vi "Pause.vi"(8 "error in (no error)":errorcluster, 11 "VICI Settings":T1) -> (0 "error out":errorcluster, 1 "Connection Error":bool, 3 "VICI Settings":T1)   [LabVIEW 2018, in "VICI M50 Party Mode.lvlib"]
uses:
  VICI M50 Party Mode.lvlib
  Settings Cluster.ctl
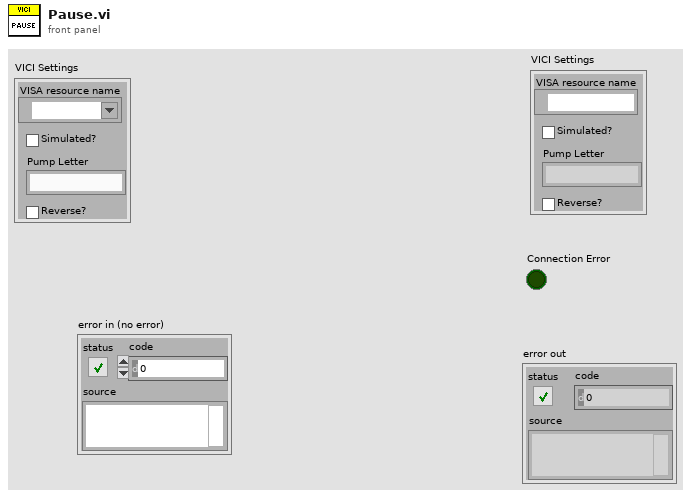
[diagram p1: front panel]
types:
  T1 = typedef "VICI M50 Party Mode.lvlib/Settings Cluster.ctl" = cluster{"VISA resource name":refnum<visa-resource-name>, "Simulated?":bool, "Pump Letter":string, "Reverse?":bool}
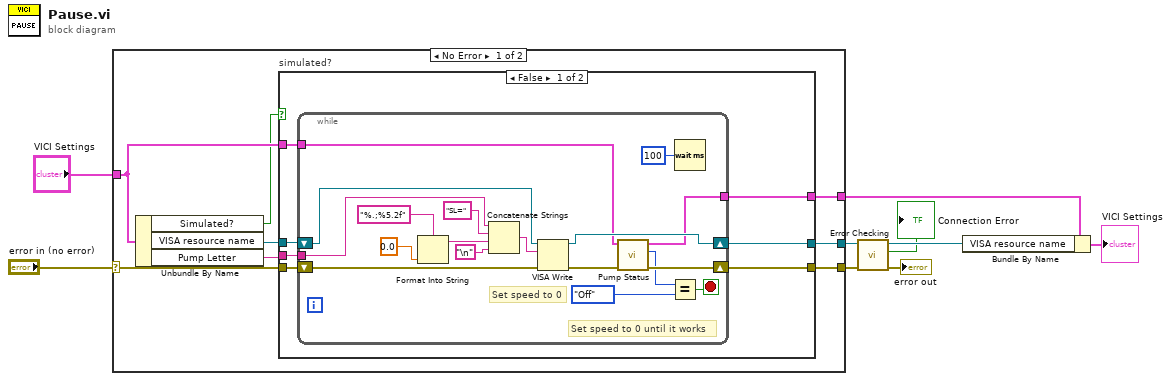
[diagram p0: block diagram]
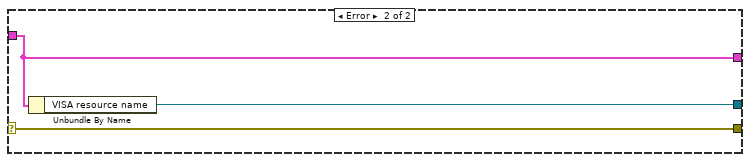
[diagram p3: hidden frame]
diagram:
  n1 = case shown="No Error" "error in (no error)" {
    selector: "error in (no error)" -> [w17 w48]
    tunnel: [w13 w47] -> w3
    tunnel: "VICI Settings" -> [w14 w47]
    tunnel: [w16 w46] -> w7
    tunnel: [w15 w48] -> w6
    frame No Error {
      n2 = Unbundle By Name(w14) -> ("Simulated?"=w11:bool, "VISA resource name"=w12:refnum<visa-resource-name>, "Pump Letter"=w10:string)
      n3 = case "simulated?" shown="False" w11 {
        tunnel: [w22 w45] -> w16
        tunnel: w12 -> [w24 w45]
        tunnel: w17 -> [w23 w44]
        tunnel: [w21 w44] -> w15
        tunnel: w14 -> [w20 w43]
        tunnel: [w19 w43] -> w13
        tunnel: w10 -> [w18 _]
        frame False {
          n4 = while {
            shift-right: [w40] -> w22
            shift-left: w24 -> [w42]
            shift-right: [w32] -> w21
            shift-left: w23 -> [w41]
            tunnel: w20 -> [w31]
            tunnel: [w30] -> w19
            tunnel: w18 -> [w25]
            stop <- w26 stop-if-true
            # "Set speed to 0 until it works"
            # "Set speed to 0"
            n5 = Format Into String(format string="%.;%5.2f", 0.0 ("input 1")) -> (resulting string=w38:string)  [unwired: 2 in, 1 out]
            n6 = Concatenate Strings(w25, "SL=" ("string"), w38, "\n") -> (w37:string)
            n7 = VISA Write(VISA resource name=w42, write buffer=w37, error in (no error)=w41) -> (VISA resource name out=w40:refnum<visa-resource-name>, error out=w33:errorcluster)  [unwired: 1 out]
            n8 = call "Pump Status.vi"("error in (no error)"=w33, "VICI Settings"=w31) -> ("error out"=w32:errorcluster, "Pump On?"=w28:enum16{"Off", "On", "Not Initialized"}, "VICI Settings"=w30:T1)  [unwired: 6 in, 1 out]
            n9 = Equal?(x=w28, y=enum16{"Off", "On", "Not Initialized"}."Off") -> (x = y?=w26:bool)
            n10 = Wait (ms)(milliseconds to wait=u32 100) -> ()  [unwired: 1 out]
          }
        }
        frame True {
        }
      }
    }
    frame Error {
      n11 = Unbundle By Name(w47) -> ("VISA resource name"=w46:refnum<visa-resource-name>)
    }
  }
  n12 = call "Error Checking.vi"("error in (no error)"=w6, "VISA resource name"=w7) -> ("error out"=→"error out":errorcluster, "Connection Error"=→"Connection Error":bool, "VISA resource name"=w4:refnum<visa-resource-name>)  [unwired: 7 in]
  n13 = Bundle By Name(cluster=w3, "VISA resource name"=w4) -> (→"VICI Settings":T1)
